vi "14_ВПОпределениеТоковВЦепи_ПримерБ.vi"() -> ()   [LabVIEW 2016]
panel:
  out "Сила тока":dynamicdata(graph)
  in  "R3":dbl
  in  "R2":dbl
  in  "R1":dbl
  in  "E":dbl
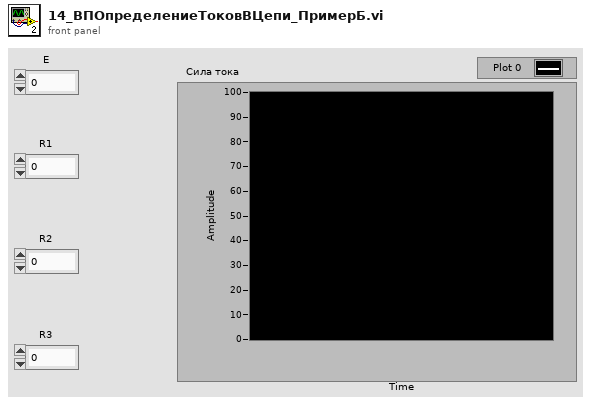
[diagram p1: front panel]
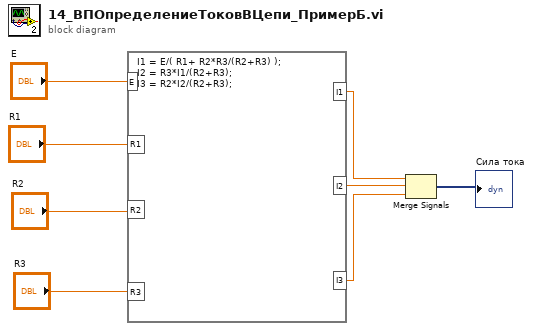
[diagram p0: block diagram]
diagram:
  n1 = formula code="I1 = E/( R1+ R2*R3/(R2+R3) );\nI2 = R3*I1/(R2+R3);\nI3 = R2*I2/(R2+R3);"("E"="E", "R1"="R1", "R2"="R2", "R3"="R3") -> ("I1"=w3:dbl, "I2"=w2:dbl, "I3"=w1:dbl)
  n2 = Merge Signals(w3, w2, w1) -> (→"Сила тока":dynamicdata)
